vi "test_broadband_noise.vi"(1 "PSD":dbl[][](array[numeric]), 2 "Sample Rate":dbl) -> (0 "HF amplitude":dbl[](array[numeric]) format="%#.2g")   [LabVIEW 2011]
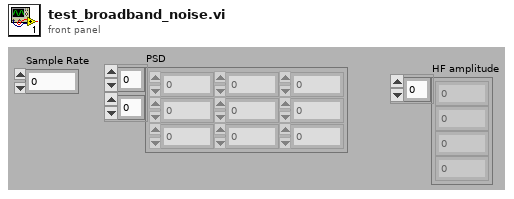
[diagram p1: front panel]
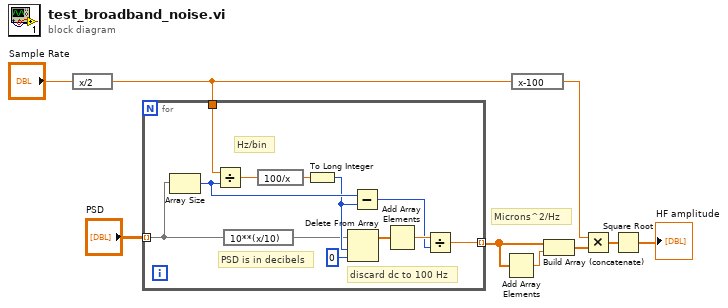
[diagram p0: block diagram]
diagram:
  # "Microns^2/Hz"
  n1 = expression code="x/2"("Sample Rate") -> (w2:dbl)
  n2 = for {
    tunnel: "PSD" -> [w12] mode=indexing
    tunnel: [w14] -> w7 mode=indexing
    tunnel: w2 -> [w13]
    # "PSD is in decibels"
    # "discard dc to 100 Hz"
    # "Hz/bin"
    n3 = Array Size(array=w12) -> (size(s)=w19:i32)
    n4 = Divide(x=w13, y=w19) -> (x/y=w17:dbl)
    n5 = expression code="10**(x/10)"(w12) -> (w11:dbl[])
    n6 = expression code="100/x"(w17) -> (w20:dbl)
    n7 = To Long Integer(number=w20) -> (32bit integer=w18:i32)
    n8 = Delete From Array(array=w11, length=w18, index=0) -> (array with subset deleted=w16:dbl[])  [unwired: 1 out]
    n9 = Subtract(x=w19, y=w18) -> (x-y=w10:i32)
    n10 = Add Array Elements(numeric array=w16) -> (sum=w15:dbl)
    n11 = Divide(x=w15, y=w10) -> (x/y=w14:dbl)
  }
  n12 = Add Array Elements(numeric array=w7) -> (sum=w8:dbl)
  n13 = expression code="x-100"(w2) -> (w1:dbl)
  n14 = Build Array (concatenate)(w7, w8) -> (w4:dbl[])
  n15 = Multiply(x=w1, y=w4) -> (x*y=w5:dbl[])
  n16 = Square Root(x=w5) -> (sqrt(x)=→"HF amplitude":dbl[])
